vi "Configure Trigger Source.vi"(8 "error in (no error)":errorcluster, 10 "trigger source":T1, 11 "VISA resource name":refnum<visa-resource-name>) -> (0 "error out":errorcluster, 3 "VISA resource name out":refnum<visa-resource-name>)   [LabVIEW 2019, in "Pulse Rider PG-1000.lvlib"]
doc: "This command queries the instrument trigger source.\n\n The trigger source can be :\n =========== ============================\n source Description\n =========== ============================\n timer internal timer\n external lock on trigger in SMA input\n manual lock on trigger key or trigger() command\n =========== ============================"
uses:
  <instrlib>/Pulse Rider PG-1000/Pulse Rider PG-1000.lvlib
  <instrlib>/Pulse Rider PG-1000/Public/Configure/Trigger/Trigger Source.ctl
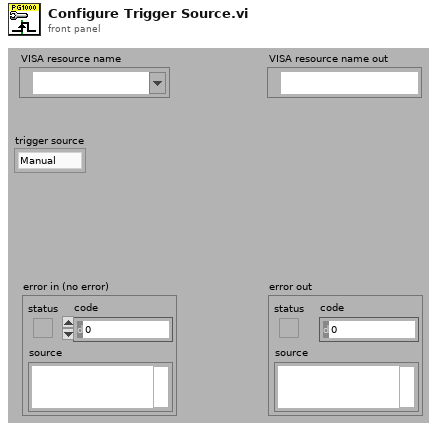
[diagram p1: front panel]
types:
  T1 = typedef "Pulse Rider PG-1000.lvlib/Trigger Source.ctl" = enum16{"Manual", "External", "Timer"}
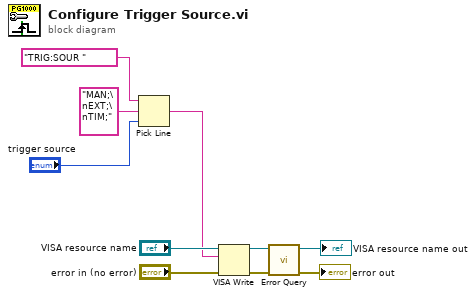
[diagram p0: block diagram]
diagram:
  n1 = Pick Line(string ("")="TRIG:SOUR ", multi-line string="MAN;\nEXT;\nTIM;" ("format string"), line index="trigger source") -> (output string=w1:string)
  n2 = VISA Write(VISA resource name="VISA resource name", write buffer=w1, error in (no error)="error in (no error)") -> (VISA resource name out=w6:refnum<visa-resource-name>, error out=w5:errorcluster)  [unwired: 1 out]
  n3 = call <instrlib>:"Error Query.vi"("error in (no error)"=w5, "VISA resource name"=w6) -> ("error out"=→"error out":errorcluster, "VISA resource name out"=→"VISA resource name out":refnum<visa-resource-name>)  [unwired: 6 in, 2 out]
